vi "Bai1_2.vi"() -> ()   [LabVIEW 2023]
panel:
  in  "stop":bool
  out "y":dbl
  out "y":dbl(slide) scale=0.0..1000.0
  out "y":dbl(knob) scale=0.0..1000.0
  out "y":dbl(knob) scale=0.0..1000.0
  out "y":dbl(knob) scale=0.0..1000.0
  out "y":dbl(knob) scale=0.0..1000.0
  in  "x":dbl
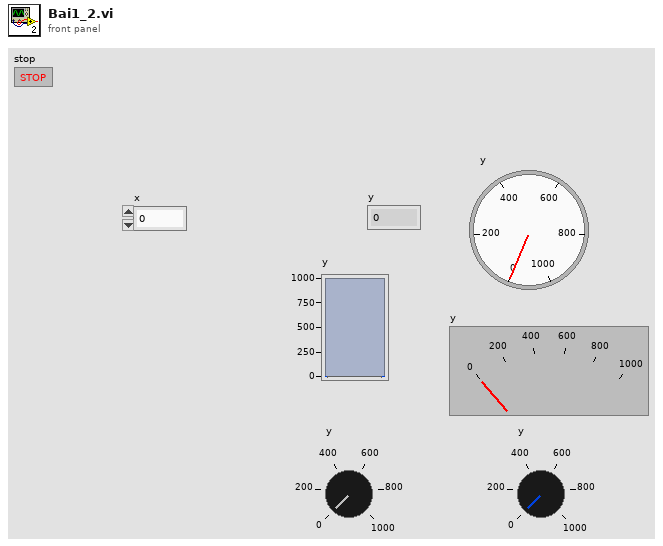
[diagram p1: front panel]
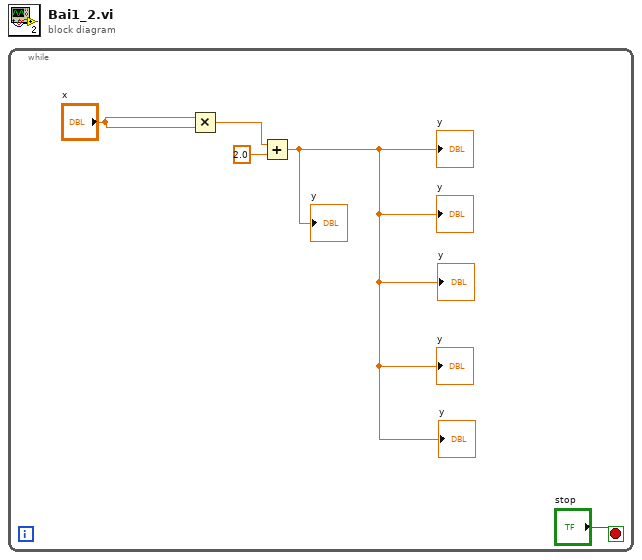
[diagram p0: block diagram]
diagram:
  n1 = while {
    stop <- "stop" stop-if-true
    n2 = Multiply(x="x", y="x") -> (x*y=w4:dbl)
    n3 = Add(x=w4, y=2.0) -> (x+y=→"y" →"y" →"y" →"y" →"y" →"y":dbl)
  }
